vi "Initialize 1553 Module.vi"(4 "debug flags (0x3000 0000)":T5={"Interrupt"=FALSE, "Initialization"=FALSE, "Module open"=FALSE, "Module close"=FALSE, "Module I/O"=FALSE, "Module recording"=FALSE, "Replay"=FALSE, "Mutex"=FALSE, "Parameter range check"=FALSE, "(internal use)"=FALSE, "Function call trace log"=FALSE, "Informational"=TRUE, "General errors"=TRUE, "Force error message box"=FALSE}, 6 "self test mode (none)":T6(ring), 8 "error in":errorcluster, 11 "device parameters":T1) -> (0 "error out":errorcluster, 3 "module handle out":u32)   [LabVIEW 2020, in "AIM MIL-STD-1553 Hardware API.lvlib"]
uses:
  AIM MIL-STD-1553 Hardware API.lvlib
  Shared/AIM Hardware Parameters.ctl
  Shared/Initialization Method.ctl
  Shared/Bus Selection.ctl
  Shared/Coupling Mode.ctl
  <instrlib>/_AIM MIL-STD-1553/PCI-1553 Mid-Level Release/1553 Utility - RT Mode Global.vi
panel:
  # "Force debug outputs related to:"
  # "log to file: aim_mil.log"
  # "e.g.: range check, etc."
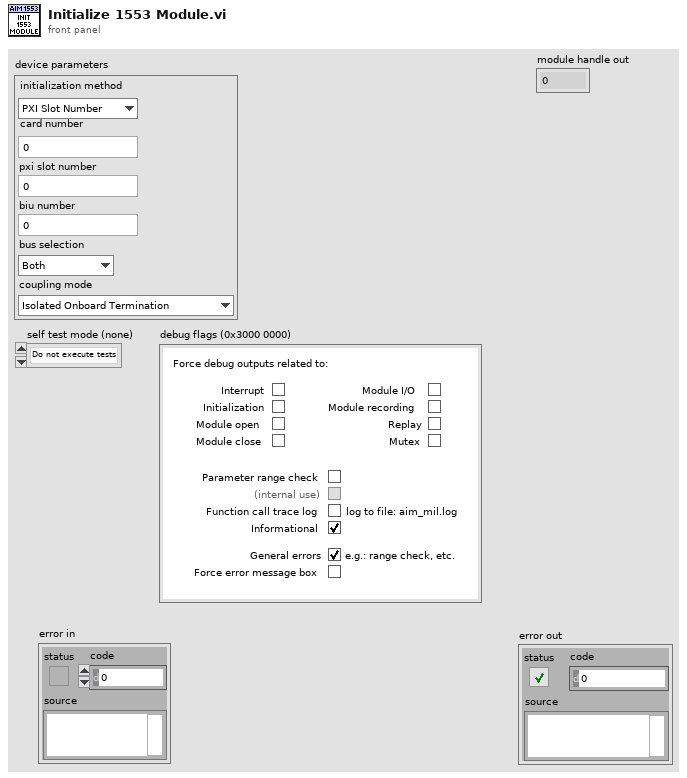
[diagram p1: front panel]
types:
  T1 = typedef "AIM Hardware Parameters.ctl" = cluster{"initialization method":T2, "card number":i32, "pxi slot number":i32, "biu number":i32, "bus selection":T3, "coupling mode":T4}
  T2 = typedef "Initialization Method.ctl" = enum16{"PXI Slot Number", "Card Number"}
  T3 = typedef "Bus Selection.ctl" = enum16{"Both", "Primary", "Secondary"}
  T4 = typedef "Coupling Mode.ctl" = enum16{"Isolated Onboard Termination", "Transformer Coupled", "Direct Coupled", "External with Onboard Termination", "Onboard Digital Wrap-around"}
  T5 = cluster{"Interrupt":bool, "Initialization":bool, "Module open":bool, "Module close":bool, "Module I/O":bool, "Module recording":bool, "Replay":bool, "Mutex":bool, "Parameter range check":bool, "(internal use)":bool, "Function call trace log":bool, "Informational":bool, "General errors":bool, "Force error message box":bool}
  T6 = enum16{"Do not execute tests", "Execute all tests", "Board enable test", "Internal self-test", "Global RAM test for BIU control block", "Global RAM test for BIU BC/RT descriptor", "Global RAM test for BIU bus monitor", "Shared RAM test from 0x100000", "Shared RAM test for CMD area", "Shared RAM test for ACK area", "Transfer test", "Interrupt test", "DAC test for bus A", "DAC test for bus B", "Timing test"}
  T7 = enum16{"Execute all tests", "Board enable test", "Internal self-test", "Global RAM test for BIU control block", "Global RAM test for BIU BC/RT descriptor", "Global RAM test for BIU bus monitor", "Shared RAM test from 0x100000", "Shared RAM test for CMD area", "Shared RAM test for ACK area", "Transfer test", "Interrupt test", "DAC test for bus A", "DAC test for bus B", "Timing test"}
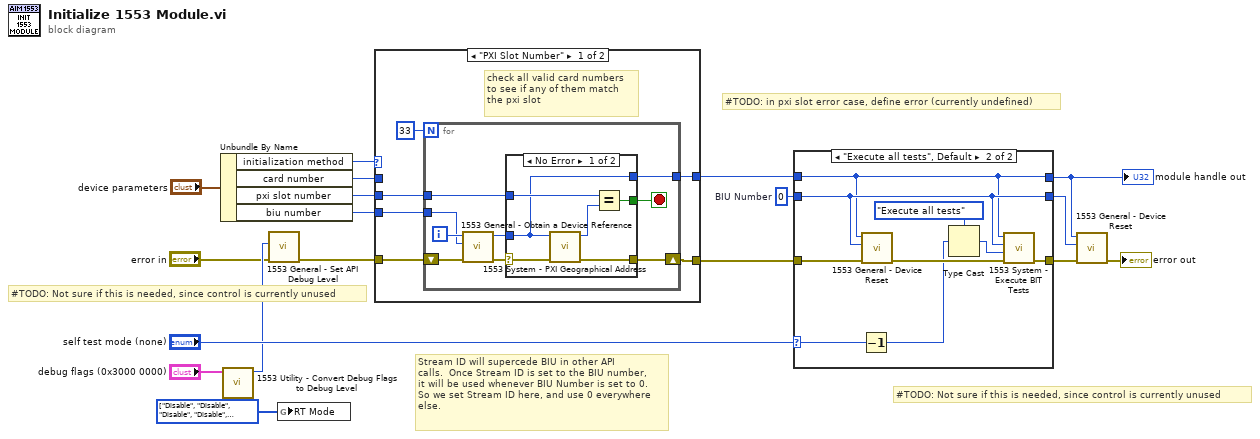
[diagram p0: block diagram]
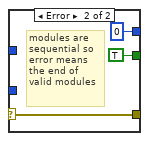
[diagram p2: hidden frame]
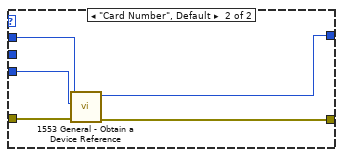
[diagram p3: hidden frame]
diagram:
  w14 = enum16{"Disable", "Simulation", "Monitor"}[] [enum."Disable", enum."Disable", enum."Disable", enum."Disable", enum."Disable", enum."Disable", enum."Disable", enum."Disable", enum."Disable", enum."Disable", enum."Disable", enum."Disable", enum."Disable", enum."Disable", enum."Disable", enum."Disable", enum."Disable", enum."Disable", enum."Disable", enum."Disable", enum."Disable", enum."Disable", enum."Disable", enum."Disable", enum."Disable", enum."Disable", enum."Disable", enum."Disable", enum."Disable", enum."Disable", enum."Disable", enum."Disable"] items=["Disable", "Simulation", "Monitor"] ("RT Mode")
  w9 = u8 0  # BIU Number
  # "Stream ID will supercede BIU in other API\ncalls.  Once Stream ID is set to the BIU number,\nit will be used whenever BIU Number is set to 0.\nSo we set Stream ID here, and use 0 everywhere\nelse."
  # "#TODO: in pxi slot error case, define error (currently undefined)"
  # "#TODO: Not sure if this is needed, since control is currently unused"
  # "#TODO: Not sure if this is needed, since control is currently unused"
  n1 = Unbundle By Name("device parameters") -> ("initialization method"=w2:T2, "card number"=w4:i32, "pxi slot number"=w1:i32, "biu number"=w3:i32)
  n2 = call <instrlib>:"1553 Utility - Convert Debug Flags to Debug Level.vi"("Debug Flags (0x3000 0000)"="debug flags (0x3000 0000)") -> ("Debug Level"=w13:u32)  [unwired: 10 in]
  n3 = call <instrlib>:"1553 General - Set API Debug Level.vi"("Error In (none)"="error in", "Debug Level (0x3000 0000)"=w13) -> ("Error Out"=w12:errorcluster)  [unwired: 9 in]
  n4 = global write "1553 Utility - RT Mode Global.vi" "RT Mode"(w14) -> ()
  n5 = case shown="\"PXI Slot Number\"" w2 {
    tunnel: w12 -> [w24 w47]
    tunnel: [w23 w46] -> w11
    tunnel: [w19 w45] -> w7
    tunnel: w4 -> [_ w44]
    tunnel: w3 -> [w21 w43]
    tunnel: w1 -> [w20 _]
    frame "PXI Slot Number" {
      # "check all valid card numbers\nto see if any of them match\nthe pxi slot"
      n6 = for {
        N: 33 -> [_]
        shift-right: [w30] -> w23
        shift-left: w24 -> [w33]
        tunnel: w21 -> [w31]
        tunnel: w20 -> [w29]
        tunnel: [w25] -> w19
        i -> [w32]
        stop <- w28 stop-if-true
        n7 = call <instrlib>:"1553 General - Obtain a Device Reference.vi"("Error In (none)"=w33, "Stream ID (1)"=w31, "Module Number (0)"=w32) -> ("Error Out"=w26:errorcluster, "Module Handle"=w27:u32)  [unwired: 7 in]
        n8 = case shown="No Error" w26 {
          selector: w26 -> [w35 w42]
          tunnel: [w39 w42] -> w30
          tunnel: w29 -> [w37 _]
          tunnel: [w36 TRUE] -> w28
          tunnel: w27 -> [w34 _]
          tunnel: [w34 u32 0 ("Module Handle")] -> w25
          frame No Error {
            n9 = call <instrlib>:"1553 System - PXI Geographical Address.vi"("Error In (none)"=w35, "Module Handle"=w34) -> ("Error Out"=w39:errorcluster, "GeographicalAddress"=w38:u32)  [unwired: 8 in]
            n10 = Equal?(x=w37, y=w38) -> (x = y?=w36:bool)
          }
          frame Error {
            # "modules are \nsequential so \nerror means \nthe end of \nvalid modules"
          }
        }
      }
    }
    frame "Card Number", Default {
      n11 = call <instrlib>:"1553 General - Obtain a Device Reference.vi"("Error In (none)"=w47, "Stream ID (1)"=w43, "Module Number (0)"=w44) -> ("Error Out"=w46:errorcluster, "Module Handle"=w45:u32)  [unwired: 7 in]
    }
  }
  n12 = case shown="\"Execute all tests\", Default" "self test mode (none)" {
    selector: "self test mode (none)" -> [_ w56]
    tunnel: w11 -> [w50 w59]
    tunnel: [w50 w57] -> w15
    tunnel: w7 -> [w48 w51]
    tunnel: w9 -> [w49 w52]
    tunnel: [w49 w52] -> w8
    tunnel: [w48 w51] -> w6
    frame "Do not execute tests" {
    }
    frame "Execute all tests", Default {
      n13 = Decrement(x=w56) -> (x-1=w55:T6)
      n14 = call <instrlib>:"1553 General - Device Reset.vi"("Error In (none)"=w59, "BIU Number (1)"=w52, "Module Handle"=w51) -> ("Error Out"=w58:errorcluster)  [unwired: 6 in, 2 out]
      n15 = Type Cast(type=T7."Execute all tests" ("Self test mode (all)"), x=w55) -> (*(type *) &x=w54:T7)
      n16 = call <instrlib>:"1553 System - Execute BIT Tests.vi"("Error In (none)"=w58, "Self test mode (all)"=w54, "BIU Number (1)"=w52, "Module Handle"=w51) -> ("Error Out"=w57:errorcluster)  [unwired: 5 in, 2 out]
    }
  }
  "module handle out" <- w6
  n17 = call <instrlib>:"1553 General - Device Reset.vi"("Error In (none)"=w15, "BIU Number (1)"=w8, "Module Handle"=w6) -> ("Error Out"=→"error out":errorcluster)  [unwired: 6 in, 2 out]
